vi "Initialize.vi"(8 "Error In":errorcluster, 11 "Draw Frame In":refnum<class "Draw Frame.lvclass">) -> (0 "Error Out":errorcluster, 3 "Draw Frame Out":refnum<class "Draw Frame.lvclass">)   [LabVIEW 2019, in "Draw Frame.lvclass"]
uses:
  Draw Frame.lvclass
  Process/Process.lvclass
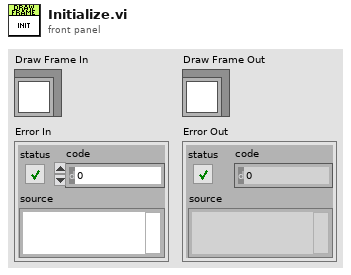
[diagram p1: front panel]
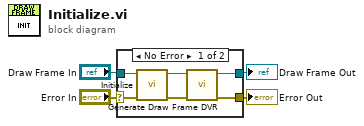
[diagram p0: block diagram]
diagram:
  n1 = case shown="No Error" "Error In" {
    selector: "Error In" -> [w10 w11]
    tunnel: [w5 w11] -> w4
    tunnel: [w6 w12] -> w3
    tunnel: "Draw Frame In" -> [w9 w12]
    frame No Error {
      n2 = call-parent "Initialize.vi"("Error In"=w10, "Process In"=w9) -> ("Error Out"=w7:errorcluster, "Process Out"=w8:refnum<class "Draw Frame.lvclass">)  [unwired: 8 in]
      n3 = call "Generate Draw Frame DVR.vi"("Error In"=w7, "Draw Frame In"=w8) -> ("Error Out"=w5:errorcluster, "Draw Frame Out"=w6:refnum<class "Draw Frame.lvclass">)  [unwired: 8 in]
    }
    frame Error {
    }
  }
  "Draw Frame Out" <- w3
  "Error Out" <- w4
